vi "7進階題-One Timer燈.vi"() -> ()   [LabVIEW 2019]
panel:
  in  "Stop":bool
  in  "Time 1":dbl=1.0 min=0.0 max=10.0 step=0.1 format="%#.1g"
  out "燈號 1":bool
  in  "按鍵 1":bool
  # "按鍵按下後，燈號依設定的時間長度ON，然後熄滅\n註：Time 1的設定區間為0~10，超出此區間，自動設成0或10；"
  # "單位：秒"
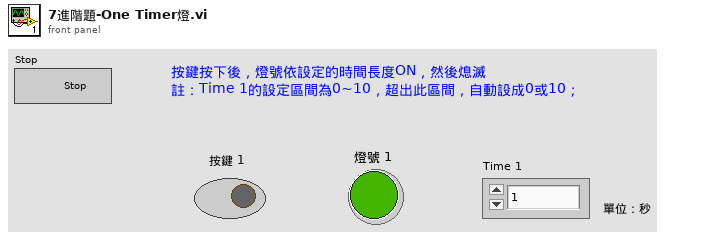
[diagram p1: front panel]
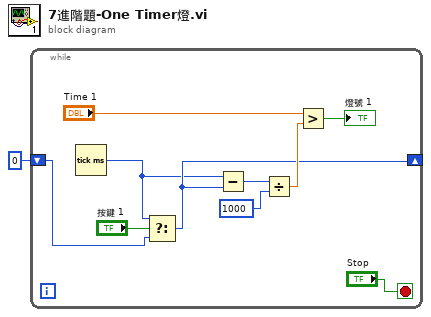
[diagram p0: block diagram]
diagram:
  n1 = while {
    shift-right: [w5] -> _
    shift-left: u32 0 ("millisecond timer value") -> [w4]
    stop <- "Stop" stop-if-true
    n2 = Tick Count (ms)() -> (millisecond timer value=w3:u32)
    n3 = Select(t=w3, s="按鍵 1", f=w4) -> (s? t:f=w5:u32)
    n4 = Subtract(x=w3, y=w5) -> (x-y=w11:u32)
    n5 = Divide(x=w11, y=u32 1000) -> (x/y=w9:dbl)
    n6 = Greater?(x="Time 1", y=w9) -> (0:→"燈號 1":bool)
  }
